vi "hw2-6 topVI.vi"() -> ()   [LabVIEW 2014]
panel:
  out "probability":dbl[](graph)
  out "number of combinations":i32[](graph)
  out "Solution":cluster{"Sum":u32, "Outcomes":dbl[][]}[](array[cluster])
  out "All outcomes":i32
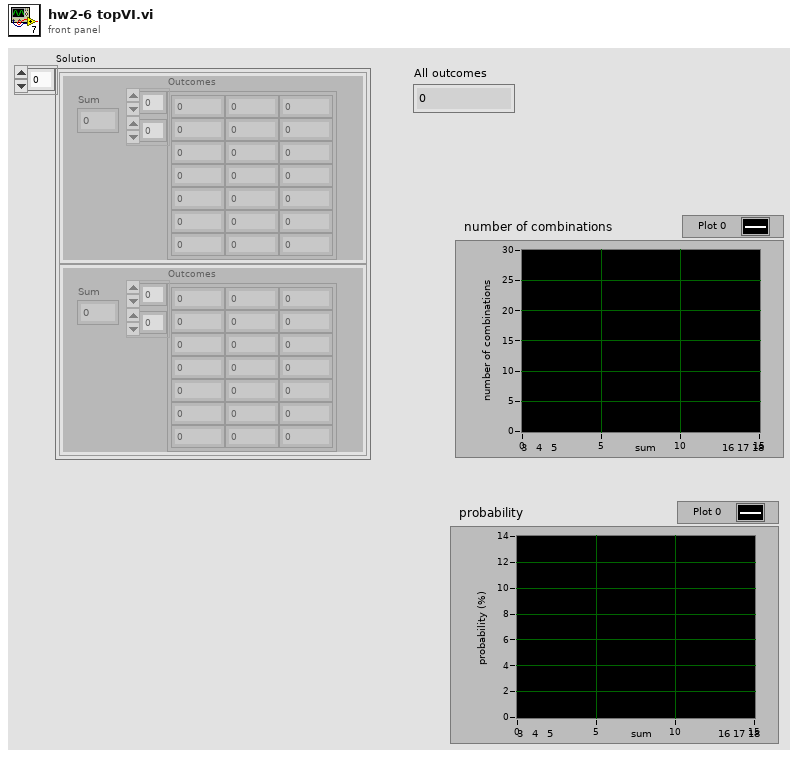
[diagram p1: front panel]
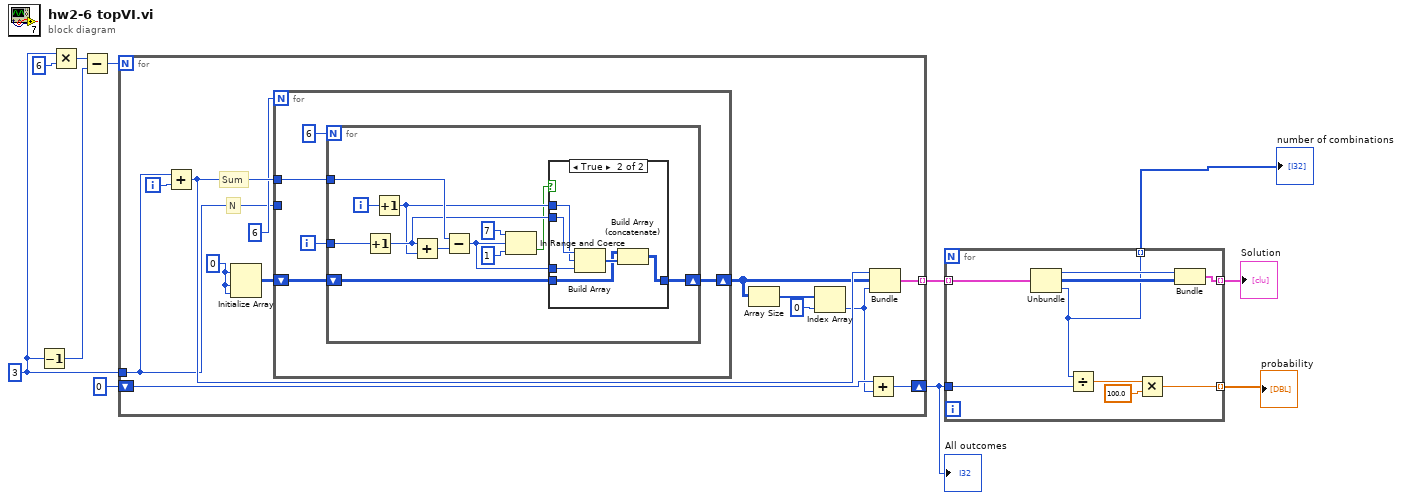
[diagram p0: block diagram]
diagram:
  w7 = 3 ("N")
  n1 = Decrement(x=w7) -> (x-1=w9:i32)
  n2 = Multiply(x=w7, y=6) -> (x*y=w10:i32)
  n3 = Subtract(x=w10, y=w9) -> (x-y=w8:i32)
  n4 = for {
    N: w8 -> [_]
    tunnel: w7 -> [w15]
    tunnel: [w17] -> w5 mode=indexing
    shift-right: [w13] -> w4
    shift-left: 0 -> [w14]
    i -> [w24]
    w22 = u32 0 ("element")
    # "Sum"
    # "N"
    n5 = Add(x=w15, y=w24) -> (x+y=w21:i32)
    n6 = Initialize Array(w22, w22, w22) -> (w23:u32[][])
    n7 = for {
      N: 6 -> [_]
      tunnel: w21 -> [w29]
      shift-right: [w26] -> w20
      shift-left: w23 -> [w27]
      tunnel: w15 -> [_]
      i -> [w28]
      n8 = for {
        N: 6 -> [_]
        tunnel: w28 -> [w40]
        tunnel: w29 -> [w39]
        shift-right: [w34] -> w26
        shift-left: w27 -> [w35]
        i -> [w41]
        n9 = Increment(x=w40) -> (x+1=w37:i32)
        n10 = Increment(x=w41) -> (x+1=w36:i32)
        n11 = Add(x=w37, y=w36) -> (x+y=w38:i32)
        n12 = Subtract(x=w39, y=w38) -> (x-y=w32:i32)
        n13 = In Range and Coerce(upper limit=7, x=w32, lower limit=1) -> (In Range?=w33:bool)  [unwired: 1 out]
        n14 = case shown="True" w33 {
          tunnel: [w42 w47] -> w34
          tunnel: w37 -> [_ w46]
          tunnel: w36 -> [_ w45]
          tunnel: w32 -> [_ w44]
          tunnel: w35 -> [w42 w43]
          frame False {
          }
          frame True {
            n15 = Build Array(w46, w45, w44) -> (w48:i32[])
            n16 = Build Array (concatenate)(w43, w48) -> (w47:u32[][])
          }
        }
      }
    }
    n17 = Array Size(array=w20) -> (size(s)=w19:i32[])
    n18 = Index Array(array=w19, index=0) -> (element=w12:i32)
    n19 = Add(x=w14, y=w12) -> (x+y=w13:i32)
    n20 = Bundle(w21, w20, w12) -> (w17:cluster{i32, u32[][], i32})  [unwired: 1 in]
  }
  "All outcomes" <- w4
  n21 = for {
    tunnel: w5 -> [w57] mode=indexing
    tunnel: w4 -> [w56]
    tunnel: [w53] -> w3 mode=indexing
    tunnel: [w50] -> w2 mode=indexing
    tunnel: [w49] -> w1 mode=indexing
    n22 = Unbundle(w57) -> (w51:i32, w55:u32[][], w50:i32)
    n23 = Divide(x=w50, y=w56) -> (x/y=w54:dbl)
    n24 = Multiply(x=w54, y=100.0) -> (x*y=w49:dbl)
    n25 = Bundle(w51, w55) -> (w53:cluster{i32, u32[][]})  [unwired: 1 in]
  }
  "Solution" <- w3
  "number of combinations" <- w2
  "probability" <- w1
